vi "Inject_Voltage.vi"(8 "error in (no error)":errorcluster, 10 "Parameters":string, 11 "reference in":refnum<class "Test_Flux_Capacitor.lvclass">) -> (0 "error out":errorcluster, 2 "Result":bool, 3 "reference out":refnum<class "Test_Flux_Capacitor.lvclass">)   [LabVIEW 2022 SP3, in "Test_Flux_Capacitor.lvlib" / "Test_Flux_Capacitor.lvclass"]
uses:
  Test_Flux_Capacitor.lvclass
  ParameterTypes/InjectVoltage.ctl
  <vilib>/Utility/error.llb/Trim Whitespace One-Sided.vi
  Components/SwitchBase.lvlibp/SwitchBase.lvclass
  Components/PSU_Base.lvlibp/PSU_Base.lvclass
  <vilib>/JDP Science/JSONtext/JSONtext.lvlib
panel:
  in  "Parameter_Type":T1
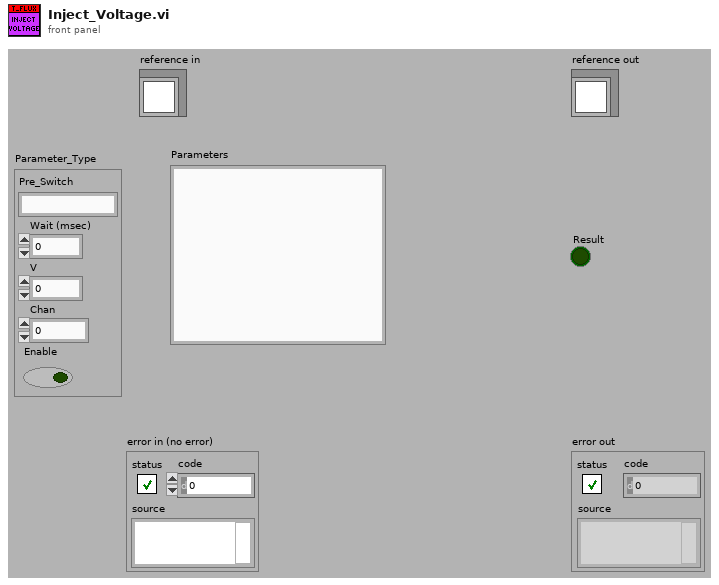
[diagram p1: front panel]
types:
  T1 = typedef "Test_Flux_Capacitor.lvlib/Test_Flux_Capacitor.lvclass/InjectVoltage.ctl" = cluster{"Pre_Switch":string, "Wait (msec)":i32, "V":dbl, "Chan":i32, "Enable":bool}
  T2 = typedef "Test_Flux_Capacitor.lvlib/Test_Flux_Capacitor.lvclass/ObjectAttributes.ctl" = cluster{"Config":T3, "DMM":refnum<class "DMM_Keysight_34980A.lvclass">, "LCR":refnum<class "LCR_BK891.lvclass">, "PSU":refnum<class "PSU_Base.lvclass">, "Switch_Manager":refnum<class "SwitchBase.lvclass">, "FRAM":string, "Flux_Capacitor":refnum<class "Flux_Capacitor.lvclass">, "Frequency_Counter":refnum<class "Frequency_Counter_Base.lvclass">, "JTAG":refnum<class "JTAG_Base.lvclass">}
  T3 = typedef "Test_Flux_Capacitor.lvlib/Test_Flux_Capacitor.lvclass/Config.ctl" = cluster{"default":string}
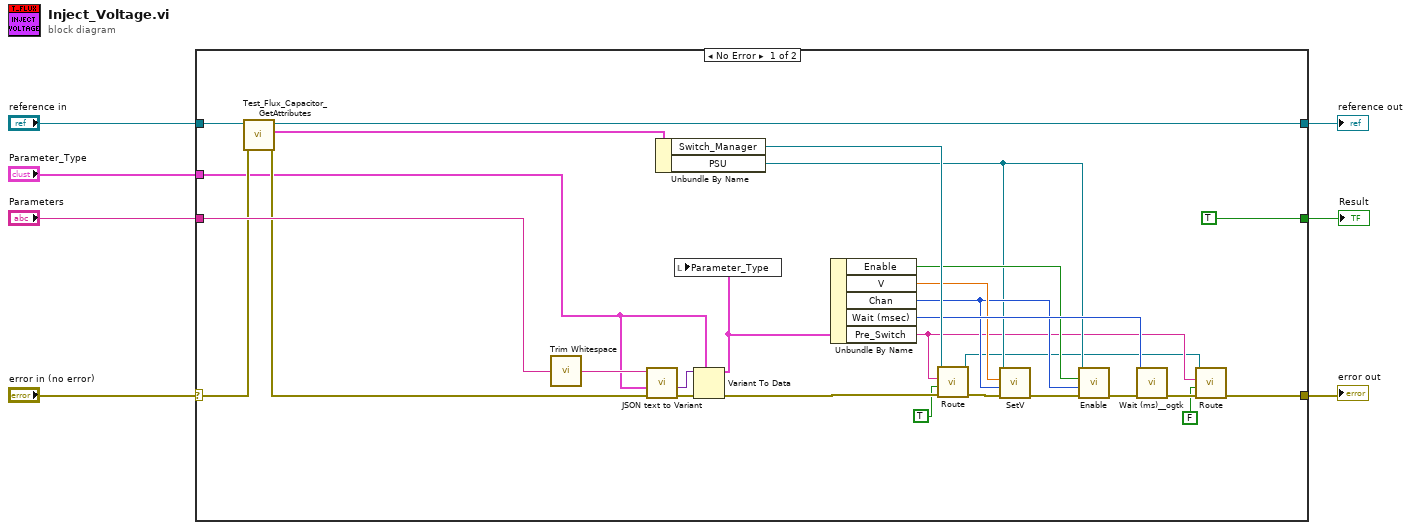
[diagram p0: block diagram]
diagram:
  n1 = case shown="No Error" "error in (no error)" {
    selector: "error in (no error)" -> [w19 w37]
    tunnel: [w11 w37] -> w6
    tunnel: [w34 w36] -> w4
    tunnel: "reference in" -> [w35 w36]
    tunnel: "Parameters" -> [w31 _]
    tunnel: "Parameter_Type" -> [w15 _]
    tunnel: [TRUE _] -> w1
    frame No Error {
      n2 = call "Test_Flux_Capacitor_GetAttributes.vi"("error in (no error)"=w19, "reference in"=w35) -> ("error out"=w18:errorcluster, "Data"=w33:T2, "reference out"=w34:refnum<class "Test_Flux_Capacitor.lvclass">)  [unwired: 6 in, 1 out]
      n3 = call <vilib>:"Trim Whitespace.vi"("string"=w31) -> ("trimmed string"=w16:string)  [unwired: 1 in]
      n4 = call <vilib>:"JSON text to Variant.vi"("error in (no error)"=w18, "Data Type"=w15, "JSON"=w16) -> ("error out"=w17:errorcluster, "Variant out"=w14:variant)  [unwired: 7 in]
      n5 = Unbundle By Name(w33) -> ("Switch_Manager"=w32:refnum<class "SwitchBase.lvclass">, "PSU"=w20:refnum<class "PSU_Base.lvclass">)
      n6 = Variant To Data(error in=w17, type=w15, Variant=w14) -> (data=w30:T1, error out=w28:errorcluster)
      n7 = local write "Parameter_Type"(w30) -> ()
      n8 = Unbundle By Name(w30) -> ("Enable"=w23:bool, "V"=w22:dbl, "Chan"=w21:i32, "Wait (msec)"=w29:i32, "Pre_Switch"=w10:string)
      n9 = call-dynamic "Route.vi"("error in (no error)"=w28, "Connect"=TRUE, "channel 1"=w10, "reference in"=w32) -> ("error out"=w26:errorcluster, "reference in"=w9:refnum<class "SwitchBase.lvclass">)  [unwired: 6 in]
      n10 = call-dynamic "SetV.vi"("error in (no error)"=w26, "Chan"=w21, "V"=w22, "reference in"=w20) -> ("error out"=w25:errorcluster)  [unwired: 6 in, 1 out]
      n11 = call-dynamic "Enable.vi"("error in (no error)"=w25, "Chan"=w21, "Enable"=w23, "reference in"=w20) -> ("error out"=w24:errorcluster)  [unwired: 6 in, 1 out]
      n12 = call <userlib>:"Wait (ms)__ogtk.vi"("error in (no error)"=w24, "milliseconds to wait"=w29) -> ("error out"=w12:errorcluster)  [unwired: 8 in, 1 out]
      n13 = call-dynamic "Route.vi"("error in (no error)"=w12, "Connect"=FALSE, "channel 1"=w10, "reference in"=w9) -> ("error out"=w11:errorcluster)  [unwired: 6 in, 1 out]
    }
    frame Error {
    }
  }
  "Result" <- w1
  "error out" <- w6
  "reference out" <- w4
